vi "Connect.vi"(8 "error in":errorcluster, 11 "4300 in":refnum<class "4300.lvclass">) -> (0 "error out":errorcluster, 3 "4300 out":refnum<class "4300.lvclass">)   [LabVIEW 2019, in "4300.lvlib" / "4300.lvclass"]
uses:
  Library/4300.lvclass
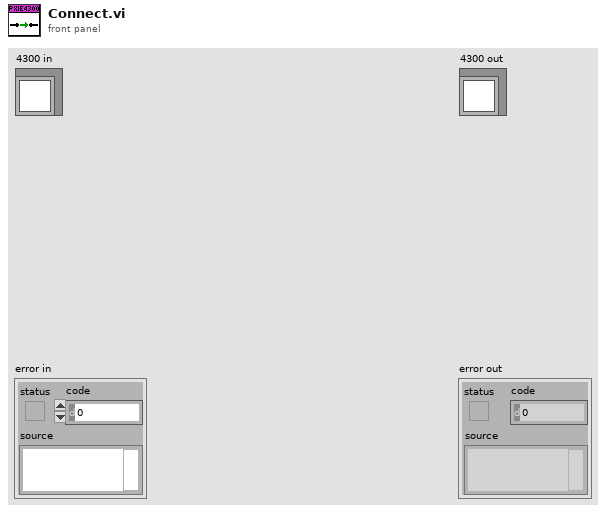
[diagram p1: front panel]
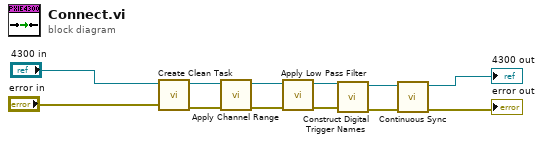
[diagram p0: block diagram]
diagram:
  n1 = call "Create Clean Task.vi"("error in"="error in", "4300 in"="4300 in") -> ("error out"=w8:errorcluster, "4300 out"=w11:refnum<class "4300.lvclass">)  [unwired: 8 in]
  n2 = call "Apply Channel Range.vi"("error in"=w8, "4300 in"=w11) -> ("error out"=w7:errorcluster, "4300 out"=w10:refnum<class "4300.lvclass">)  [unwired: 8 in]
  n3 = call "Apply Low Pass Filter.vi"("error in"=w7, "4300 in"=w10) -> ("error out"=w5:errorcluster, "4300 out"=w6:refnum<class "4300.lvclass">)  [unwired: 8 in]
  n4 = call "Construct Digital Trigger Names.vi"("error in"=w5, "4300 in"=w6) -> ("error out"=w3:errorcluster, "4300 out"=w4:refnum<class "4300.lvclass">)  [unwired: 8 in]
  n5 = call "Continuous Sync.vi"("error in"=w3, "4300 in"=w4) -> ("error out"=→"error out":errorcluster, "4300 out"=→"4300 out":refnum<class "4300.lvclass">)  [unwired: 8 in]
